vi "poly_is_running_ref.vi"(4 "vi ref":refnum<vi>) -> (1 "state = 'Running'?":bool)   [LabVIEW 2015]
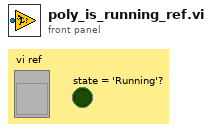
[diagram p1: front panel]
types:
  T1 = enum32{"Bad", "Idle", "Run top level", "Running"}
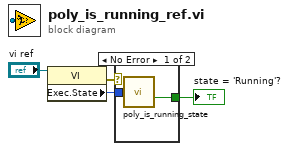
[diagram p0: block diagram]
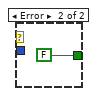
[diagram p2: hidden frame]
diagram:
  n1 = property class="VI"(reference="vi ref") -> (error out=w1:errorcluster, "Exec.State"=w3:T1)  [unwired: 1 in, 1 out]
  n2 = case shown="No Error" w1 {
    tunnel: w3 -> [w6 _]
    tunnel: [w5 FALSE] -> w2
    frame No Error {
      n3 = call "poly_is_running_state.vi"("execution state"=w6) -> ("state = 'Running'?"=w5:bool)  [unwired: 4 in]
    }
    frame Error {
    }
  }
  "state = 'Running'?" <- w2
